vi "Self-Test.vi"(8 "error in (no error)":errorcluster, 11 "3446X in":refnum<class "3446X.lvclass">) -> (0 "error out":errorcluster, 1 "Self-Test Message":string, 2 "Self-Test Result (Pass=T)":bool, 3 "3446X out":refnum<class "3446X.lvclass">)   [LabVIEW 2018, in "3446X.lvlib" / "3446X.lvclass"]
uses:
  3446X.lvclass
  3446X.lvclass/3446X.ctl
  <instrlib>/Agilent 3446X Series/Agilent 3446X Series.lvlib
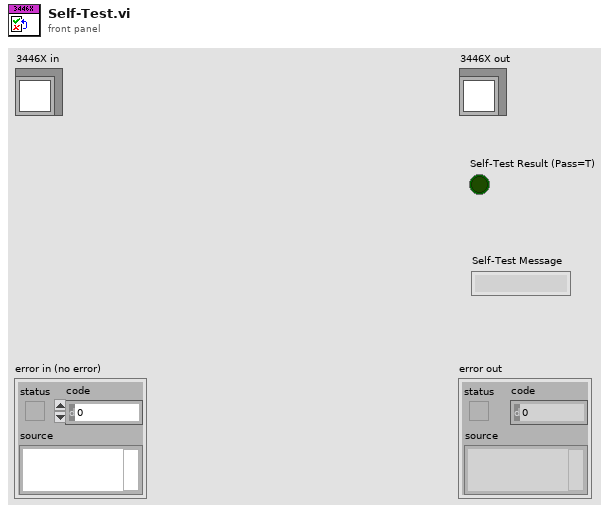
[diagram p1: front panel]
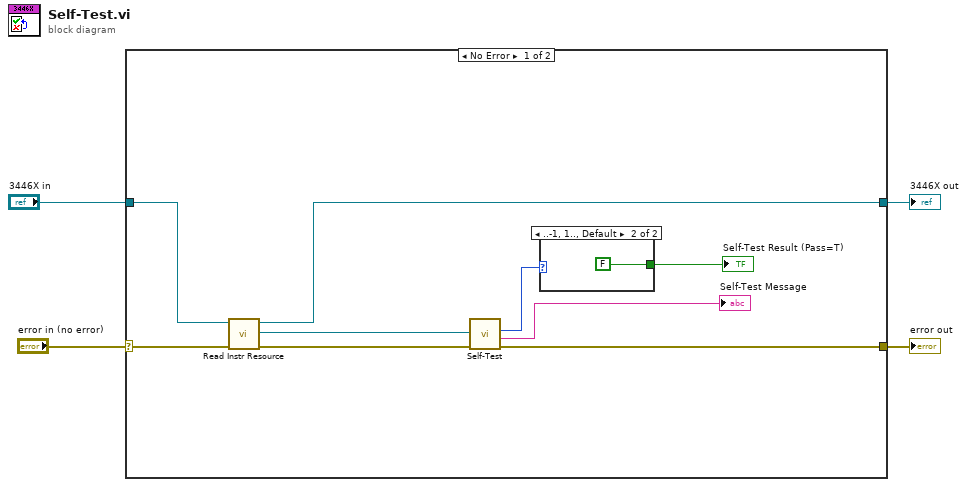
[diagram p0: block diagram]
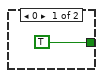
[diagram p2: hidden frame]
diagram:
  n1 = case shown="No Error" "error in (no error)" {
    selector: "error in (no error)" -> [w13 w16]
    tunnel: "3446X in" -> [w12 w17]
    tunnel: [w11 w17] -> w2
    tunnel: [w7 w16] -> w1
    frame No Error {
      n2 = call "Read Instr Resource.vi"("error in (no error)"=w13, "3446X in"=w12) -> ("error out"=w9:errorcluster, "Instr Resource"=w10:refnum<visa-resource-name>, "3446X out"=w11:refnum<class "3446X.lvclass">)  [unwired: 7 in]
      n3 = call <instrlib>:"Self-Test.vi"("error in (no error)"=w9, "VISA resource name"=w10) -> ("error out"=w7:errorcluster, "Self-Test Result Message"=→"Self-Test Message":string, "Self-Test Result Code"=w6:i32)  [unwired: 6 in, 1 out]
      n4 = case shown="..-1, 1.., Default" w6 {
        tunnel: [TRUE FALSE] -> w5
        frame 0 {
        }
        frame ..-1, 1.., Default {
        }
      }
      "Self-Test Result (Pass=T)" <- w5
    }
    frame Error {
    }
  }
  "error out" <- w1
  "3446X out" <- w2
